vi "盐度补偿值读取.vi"(8 "Error in":errorcluster caption="Error in (no error)", 11 "MB session in":refnum<class "MB_Master.lvclass">) -> (0 "error out":errorcluster, 2 "盐度补偿值":sgl, 3 "MB session out":refnum<class "MB_Master.lvclass">)   [LabVIEW 2016, in "斯坦道氟化物.lvlib"]
uses:
  <vilib>/Plasmionique/MB Master/MB_Master/MB_Master.lvclass
  <vilib>/Plasmionique/MB Master/MB Master.lvlib
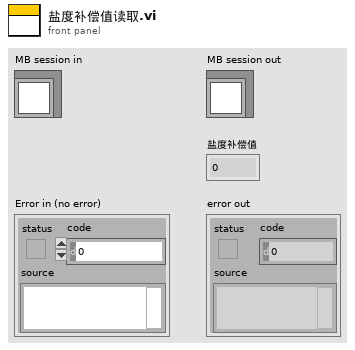
[diagram p1: front panel]
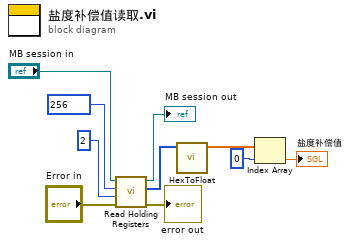
[diagram p0: block diagram]
diagram:
  n1 = call <vilib>:"Read Holding Registers.vi"("error in (no error)"="Error in", "quantity"=u16 2, "starting address"=u16 256, "MB session in"="MB session in") -> ("error out"=→"error out":errorcluster, "Registers"=w4:u16[], "MB session out"=→"MB session out":refnum<class "MB_Master.lvclass">)  [unwired: 5 in]
  n2 = call "HexToFloat.vi"("数组"=w4) -> ("FLOAT"=w3:sgl[])  [unwired: 10 in]
  n3 = Index Array(array=w3, index=0 ("索引")) -> (element=→"盐度补偿值":sgl)
